vi "Example Callback 2.vi"() -> ()   [LabVIEW 2010]
uses:
  C:/tf/play/labview/Tinkerforge.dll
  Tinkerforge.dll
panel:
  out "temperature (°C)":sgl format="%#_13g"
  in  "stop":bool
  out "humidity (%RH)":sgl format="%#_13g"
  in  "uid":string="Dkq"
  in  "port":i32=4223
  in  "host":string="localhost"
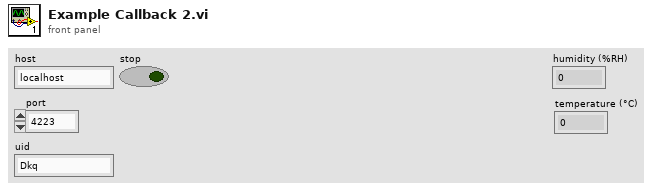
[diagram p1: front panel]
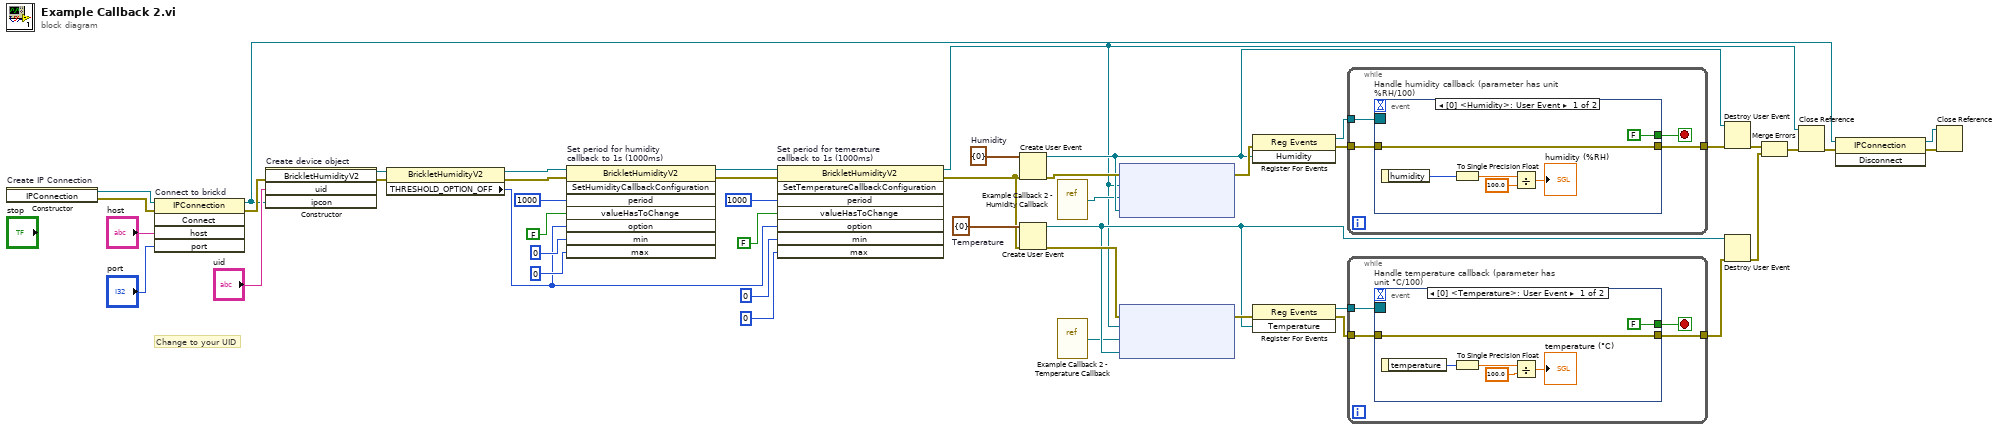
[diagram p0: block diagram]
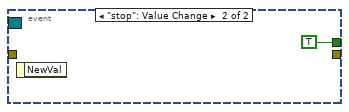
[diagram p2: hidden frame]
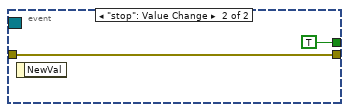
[diagram p3: hidden frame]
diagram:
  w14 = cluster{"temperature":i16} {"temperature"=0}  # Temperature
  w31 = cluster{"humidity":i32} {"humidity"=0}  # Humidity
  # "Change to your UID"
  n1 = constructor on="Create IP Connection" class="IPConnection"() -> (reference out=w46:refnum<k24>, error out=w29:errorcluster)  [unwired: 3 in, 1 out]
  n2 = invoke on="Connect to brickd" class="IPConnection" method="Connect"(reference=w46, error in=w29, "host"="host", "port"="port") -> (reference out=w39:refnum<k24>, error out=w42:errorcluster)  [unwired: 1 in, 3 out]
  n3 = constructor on="Create device object" class="BrickletHumidityV2"(error in=w42, "uid"="uid", "ipcon"=w39) -> (reference out=w25:refnum<k24>, error out=w23:errorcluster)  [unwired: 2 in, 3 out]
  n4 = property class="BrickletHumidityV2"(reference=w25, error in=w23) -> (reference out=w24:refnum<k24>, error out=w22:errorcluster, "THRESHOLD_OPTION_OFF"=w8:u16)
  n5 = invoke on="Set period for humidity\ncallback to 1s (1000ms)" class="BrickletHumidityV2" method="SetHumidityCallbackConfiguration"(reference=w24, error in=w22, "period"=i64 1000, "valueHasToChange"=FALSE, "option"=w8, "min"=0, "max"=0) -> (reference out=w3:refnum<k24>, error out=w5:errorcluster)  [unwired: 1 in, 6 out]
  n6 = invoke on="Set period for temerature\ncallback to 1s (1000ms)" class="BrickletHumidityV2" method="SetTemperatureCallbackConfiguration"(reference=w3, error in=w5, "period"=i64 1000, "valueHasToChange"=FALSE, "option"=w8, "min"=i16 0, "max"=i16 0) -> (reference out=w2:refnum<k24>, error out=w4:errorcluster)  [unwired: 1 in, 6 out]
  n7 = Create User Event(user event datatype=w31, error in=w4) -> (user event=w32:refnum<user-event>, error out=w37:errorcluster)
  n8 = Create User Event(user event datatype=w14, error in=w4) -> (user event=w15:refnum<user-event>, error out=w20:errorcluster)
  n9 = vi-ref "Example Callback 2 - Humidity Callback.vi"() -> ("vi reference"=w21:refnum<vi>)
  n10 = vi-ref "Example Callback 2 - Temperature Callback.vi"() -> ("vi reference"=w1:refnum<vi>)
  n11 = node ("Register Event Callback")(w37, w2, w21, w32) -> (w36:errorcluster)  [unwired: 1 in, 1 out]
  n12 = node ("Register Event Callback")(w20, w2, w1, w15) -> (w19:errorcluster)  [unwired: 1 in, 1 out]
  n13 = register-events(error in=w36, w32) -> (reference out=w35:refnum<event-registration>, error out=w33:errorcluster)  [unwired: 1 in]
  n14 = register-events(error in=w19, w15) -> (reference out=w18:refnum<event-registration>, error out=w16:errorcluster)  [unwired: 1 in]
  n15 = while {
    tunnel: w35 -> [w50]
    tunnel: [w49] -> w34
    tunnel: w33 -> [w48]
    stop <- w47 stop-if-true
    n16 = event "Handle humidity callback (parameter has unit %RH/100)" shown="[0] <Humidity>: User Event" {
      selector: w50 -> [_ _]
      dyn-events: _ -> [_ _]
      timeout: _ -> [_ _]
      tunnel: [w53 w57] -> w49
      tunnel: w48 -> [w53 w57]
      tunnel: [FALSE TRUE] -> w47
      event User Event {
        n17 = event-data() -> ("humidity"=w54:i32)  [unwired: 1 in]
        n18 = To Single Precision Float(number=w54) -> (single precision float=w55:sgl)
        n19 = Divide(x=w55, y=sgl 100.0) -> (x/y=→"humidity (%RH)":sgl)
      }
      event "stop": Value Change {
        n20 = event-data() -> ()  [unwired: 1 in, 1 out]
      }
    }
  }
  n21 = while {
    tunnel: w18 -> [w62]
    tunnel: [w61] -> w17
    tunnel: w16 -> [w60]
    stop <- w59 stop-if-true
    n22 = event "Handle temperature callback (parameter has unit °C/100)" shown="[0] <Temperature>: User Event" {
      selector: w62 -> [_ _]
      dyn-events: _ -> [_ _]
      timeout: _ -> [_ _]
      tunnel: [w65 _] -> w61
      tunnel: w60 -> [w65 _]
      tunnel: [FALSE TRUE] -> w59
      event User Event {
        n23 = event-data() -> ("temperature"=w66:i16)  [unwired: 1 in]
        n24 = To Single Precision Float(number=w66) -> (single precision float=w67:sgl)
        n25 = Divide(x=w67, y=sgl 100.0) -> (x/y=→"temperature (°C)":sgl)
      }
      event "stop": Value Change {
        n26 = event-data() -> ()  [unwired: 1 in, 1 out]
      }
    }
  }
  n27 = Destroy User Event(user event=w32, error in=w34) -> (error out=w13:errorcluster)
  n28 = Destroy User Event(user event=w15, error in=w17) -> (error out=w11:errorcluster)
  n29 = Merge Errors(w13, w11) -> (w12:errorcluster)
  n30 = Close Reference(reference=w2, error in (no error)=w12) -> (error out=w41:errorcluster)
  n31 = invoke class="IPConnection" method="Disconnect"(reference=w39, error in=w41) -> (reference out=w38:refnum<k24>, error out=w40:errorcluster)  [unwired: 1 in, 1 out]
  n32 = Close Reference(reference=w38, error in (no error)=w40) -> ()  [unwired: 1 out]
